vi "Initialise.vi"(8 "error in (no error)":errorcluster, 10 "Message in":refnum<class "InitialiseMessage.lvclass">, 11 "Tomo in":refnum<class "Tomo.lvclass">) -> (0 "error out":errorcluster, 3 "Tomo out":refnum<class "Tomo.lvclass">)   [LabVIEW 2012, in "Tomo.lvclass"]
doc: "This method is called when an initialise message is received. It mainly initialises the RabbitMQ connectivity. \n\nOverride this method when your component needs special initialisation (e.g. of software or hardware resources). In that case, don't forget to call the parent for proper implementation. If your component owns subcomponents, they count as resources, so you have to initialise them by calling their own initialise functions"
uses:
  Tomo.lvclass
  <vilib>/Distrio/Murmex/InitialiseMessage/InitialiseMessage.lvclass
  <vilib>/Distrio/Murmex/Murmex/Murmex.lvclass
  Current activity.ctl
  Tomo.lvclass/Tomo.ctl
panel:
  # "This method is called when the INTIALISE\ntrigger is sent. \n\nOverride this method when your component needs to\nrespond to this trigger. \n\nCall parent for proper implementation"
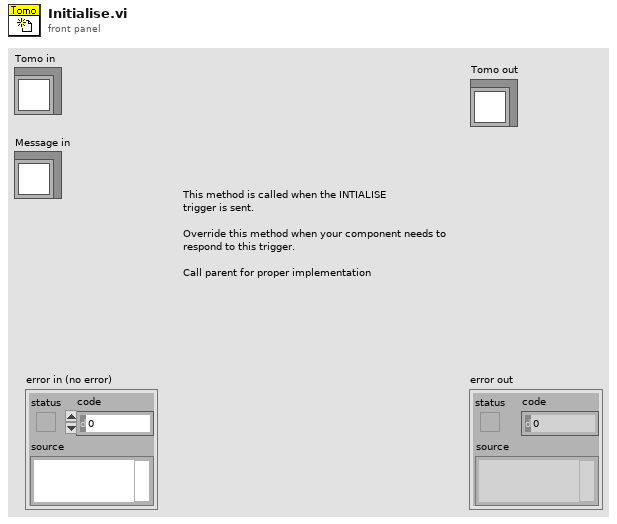
[diagram p1: front panel]
types:
  T1 = typedef "Tomo.lvclass/Current activity.ctl" = enum16{"Idle", "Inter-stack motion", "Pre-tomo calculation", "Stack acquisition", "Stack preparation", "Pre-tomo stack acq", "Pre-tomo inter-stack"}
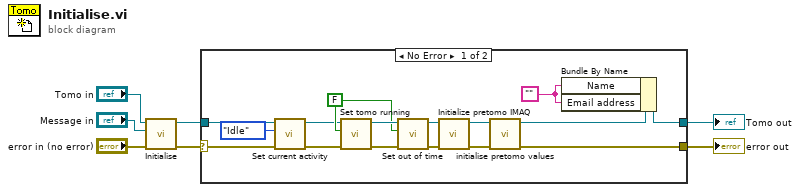
[diagram p0: block diagram]
diagram:
  n1 = call-parent "Initialise.vi"("error in (no error)"="error in (no error)", "Message in"="Message in", "Murmex in"="Tomo in") -> ("error out"=w4:errorcluster, "Murmex out"=w3:refnum<class "Tomo.lvclass">)  [unwired: 7 in]
  n2 = case shown="No Error" w4 {
    selector: w4 -> [w17 w24]
    tunnel: w3 -> [w18 w25]
    tunnel: [w11 w24] -> w2
    tunnel: [w9 w25] -> w1
    frame No Error {
      w8 = ""
      w21 = FALSE ("is acquiring?")
      n3 = call-dynamic "Set current activity.vi"("error in (no error)"=w17, "Current activity"=Current_activity."Idle", "Tomo in"=w18) -> ("error out"=w19:errorcluster, "Tomo out"=w20:refnum<class "Tomo.lvclass">)  [unwired: 7 in]
      n4 = call-dynamic "Set tomo running.vi"("error in (no error)"=w19, "tomo running?"=w21, "Tomo in"=w20) -> ("error out"=w23:errorcluster, "Tomo out"=w22:refnum<class "Tomo.lvclass">)  [unwired: 7 in]
      n5 = call-dynamic "Set out of time.vi"("error in (no error)"=w23, "out of time?"=w21, "Tomo in"=w22) -> ("error out"=w15:errorcluster, "Tomo out"=w14:refnum<class "Tomo.lvclass">)  [unwired: 7 in]
      n6 = call-dynamic "Initialize pretomo IMAQ.vi"("error in (no error)"=w15, "Tomo in"=w14) -> ("error out"=w12:errorcluster, "Tomo out"=w13:refnum<class "Tomo.lvclass">)  [unwired: 8 in]
      n7 = call-dynamic "initialise pretomo values.vi"("error in (no error)"=w12, "Tomo in"=w13) -> ("error out"=w11:errorcluster, "Tomo out"=w10:refnum<class "Tomo.lvclass">)  [unwired: 8 in]
      n8 = Bundle By Name(cluster=w10, "Name"=w8, "Email address"=w8) -> (w9:refnum<class "Tomo.lvclass">)
    }
    frame Error {
    }
  }
  "error out" <- w2
  "Tomo out" <- w1
